vi "file - read-write - list of lines.vi"(7 "read/write control":T1, 9 "header":string, 10 "list of lines IN":string[](array[string]), 11 "file path":path=path "\\\\rus-one\\newdata/data/Ultrasound/Experiment/ProbeTest/Probe10/Hg1201-6-C185-550Cair-3c-83K/sweep3/9w/3366_a.dat") -> (1 "header OUT":string, 2 "list of lines OUT":string[](array[string]), 3 "filename out":string)   [LabVIEW 2020]
uses:
  file -- read-write control.ctl
  <vilib>/Utility/file.llb/Read Delimited Spreadsheet (string).vi
  <vilib>/Utility/file.llb/Write Delimited Spreadsheet (string).vi
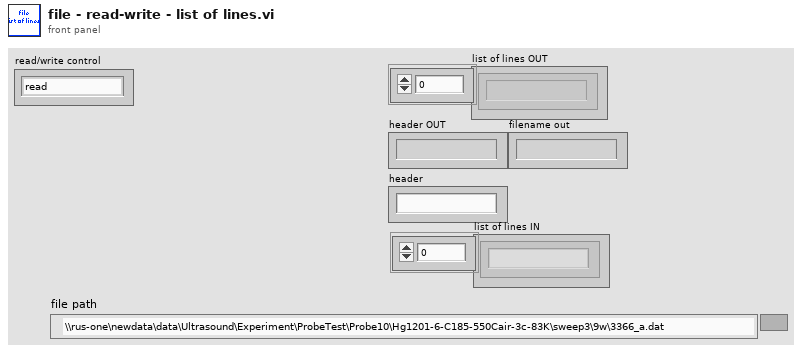
[diagram p1: front panel]
types:
  T1 = typedef "file -- read-write control.ctl" = enum16{"read", "write all", "append one line"}
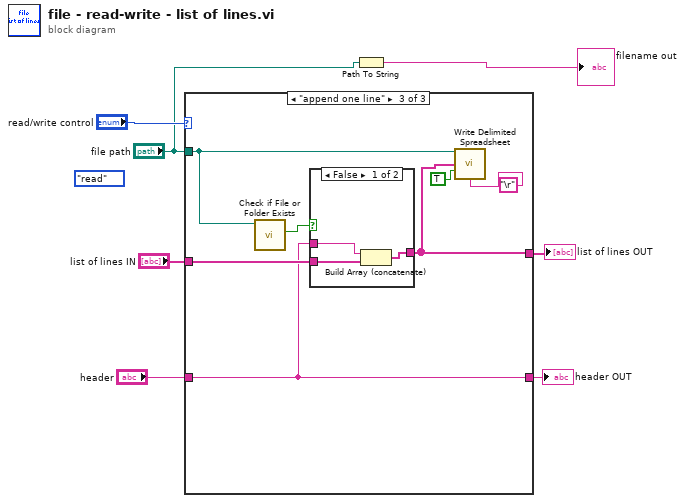
[diagram p0: block diagram]
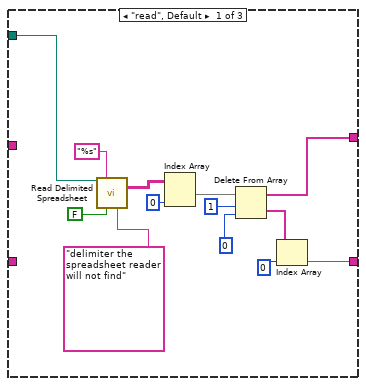
[diagram p2: hidden frame]
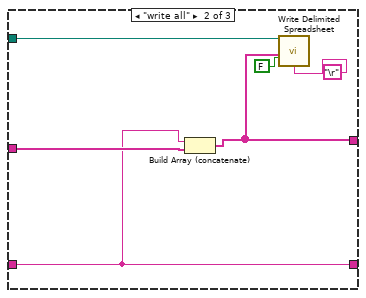
[diagram p3: hidden frame]
diagram:
  (unwired) file_--_read-write_control."read" ("read/write control")
  n1 = case shown="\"append one line\"" "read/write control" {
    tunnel: "file path" -> [w13 w24 w30]
    tunnel: [w9 w21 w27] -> w7
    tunnel: [w8 w22 w28] -> w6
    tunnel: "header" -> [_ w22 w28]
    tunnel: "list of lines IN" -> [_ w23 w29]
    frame "read", Default {
      n2 = call-poly <vilib>:"Read Delimited Spreadsheet.vi"("file path (dialog if empty)"=w13, "format (%s)"="%s", "transpose? (F)"=FALSE ("append to file? (new file:F)"), "delimiter (\\t)"="delimiter the spreadsheet reader will not find" ("delimiter (\\t)")) -> ("all rows"=w18:string[][])  [unwired: 6 in, 5 out]
      n3 = Index Array(array=w18, index (col)=0 ("disabled index (col)")) -> (element=w16:string[])  [unwired: 1 in]
      n4 = Delete From Array(array=w16, length=1, index=0) -> (deleted portion=w11:string[], array with subset deleted=w9:string[])
      n5 = Index Array(array=w11, index=0 ("disabled index (col)")) -> (element=w8:string)
    }
    frame "write all" {
      n6 = Build Array (concatenate)(w22, w23) -> (w21:string[])
      n7 = call-poly <vilib>:"Write Delimited Spreadsheet.vi"("file path (dialog if empty)"=w24, "1D data"=w21, "append to file? (new file:F)"=FALSE, "delimiter (\\t)"="\r") -> ()  [unwired: 10 in, 2 out]
    }
    frame "append one line" {
      n8 = call <vilib>:"Check if File or Folder Exists.vi"("path"=w30) -> ("file or folder exists?"=w31:bool)  [unwired: 8 in, 2 out]
      n9 = case shown="False" w31 {
        tunnel: w29 -> [w36 w37]
        tunnel: w28 -> [w35 _]
        tunnel: [w34 w37] -> w27
        frame False {
          n10 = Build Array (concatenate)(w35, w36) -> (w34:string[])
        }
        frame True {
        }
      }
      n11 = call-poly <vilib>:"Write Delimited Spreadsheet.vi"("file path (dialog if empty)"=w30, "1D data"=w27, "append to file? (new file:F)"=TRUE, "delimiter (\\t)"="\r") -> ()  [unwired: 10 in, 2 out]
    }
  }
  "list of lines OUT" <- w7
  "header OUT" <- w6
  n12 = Path To String(path="file path") -> (string=→"filename out":string)
